vi "getCenterpt.vi"(4 "markers3":dbl[](array[numeric])) -> (0 "centerxyz":dbl[](array[numeric]))   [LabVIEW 2024]
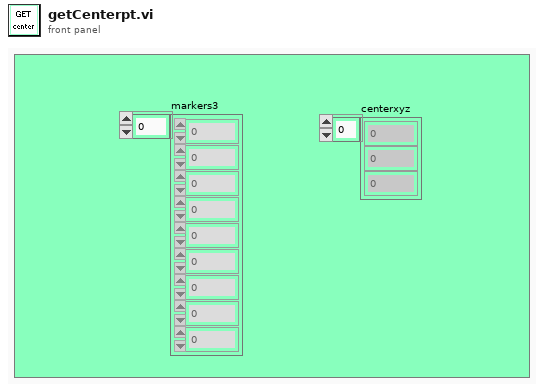
[diagram p1: front panel]
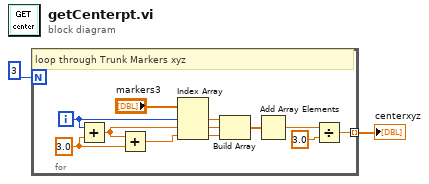
[diagram p0: block diagram]
diagram:
  n1 = for {
    N: 3 -> [_]
    tunnel: [w3] -> w1 mode=indexing
    i -> [w14]
    w12 = 3.0 ("y")
    # "loop through Trunk Markers xyz"
    n2 = Add(x=w14, y=w12) -> (x+y=w13:dbl)
    n3 = Add(x=w13, y=w12) -> (x+y=w11:dbl)
    n4 = Index Array(array="markers3", index #1=w14, index #2=w13, index #3=w11) -> (element #1=w9:dbl, element #2=w8:dbl, element #3=w7:dbl)
    n5 = Build Array(w9, w8, w7) -> (w6:dbl[])
    n6 = Add Array Elements(numeric array=w6) -> (sum=w5:dbl)
    n7 = Divide(x=w5, y=3.0) -> (x/y=w3:dbl)
  }
  "centerxyz" <- w1
